vi "BenchmarkSorting.vi"() -> ()   [LabVIEW 2014]
panel:
  out "Bubble Sort(ms)":u32
  out "Insertion Sort(ms)":u32
  out "Selection Sort(ms)":u32
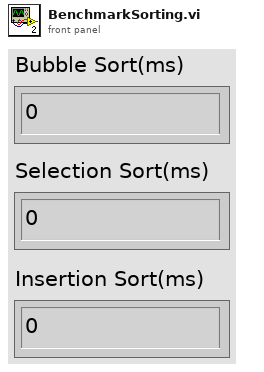
[diagram p1: front panel]
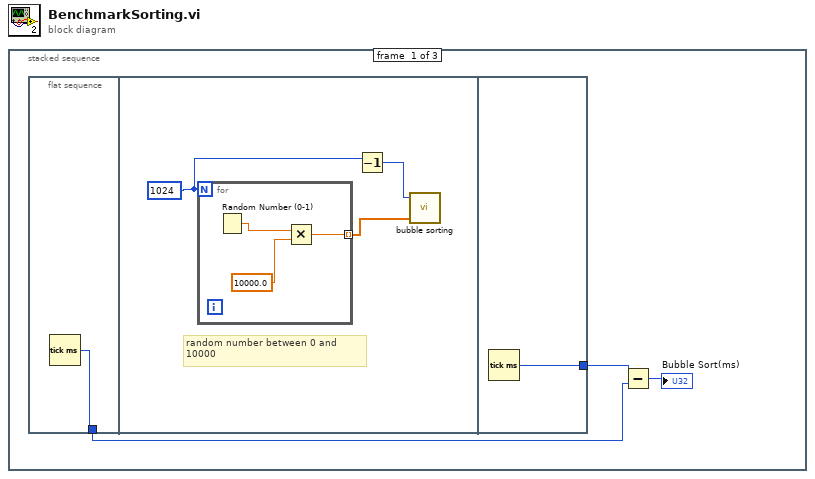
[diagram p0: block diagram]
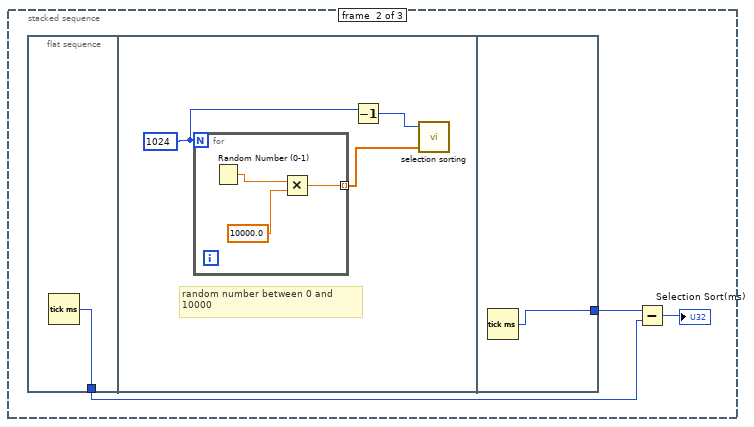
[diagram p2: hidden frame]
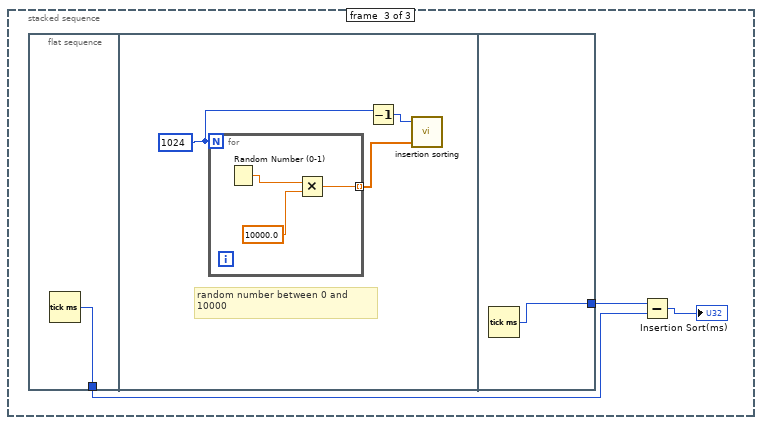
[diagram p3: hidden frame]
diagram:
  n1 = stacked-sequence {
    frame #0 {
      n2 = flat-sequence {
        tunnel: [w4] -> _
        tunnel: [w4] -> w2
        tunnel: [w11] -> w3
        frame #0 {
          n3 = Tick Count (ms)() -> (millisecond timer value=w4:u32)
        }
        frame #1 {
          w7 = 1024
          # "random number between 0 and\n10000"
          n4 = for {
            N: w7 -> [_]
            tunnel: [w8] -> w5 mode=indexing
            n5 = Random Number (0-1)() -> (number: 0 to 1=w10:dbl)
            n6 = Multiply(x=w10, y=10000.0) -> (x*y=w8:dbl)
          }
          n7 = Decrement(x=w7) -> (x-1=w6:i32)
          n8 = call "bubble sorting.vi"("value between1~10000"=w5, "N numbers"=w6) -> ()  [unwired: 3 in]
        }
        frame #2 {
          n9 = Tick Count (ms)() -> (millisecond timer value=w11:u32)
        }
      }
      n10 = Subtract(x=w3, y=w2) -> (x-y=→"Bubble Sort(ms)":u32)
    }
    frame #1 {
      n11 = flat-sequence {
        tunnel: [w15] -> w13
        tunnel: [w22] -> w14
        frame #0 {
          n12 = Tick Count (ms)() -> (millisecond timer value=w15:u32)
        }
        frame #1 {
          w18 = 1024
          # "random number between 0 and\n10000"
          n13 = for {
            N: w18 -> [_]
            tunnel: [w19] -> w16 mode=indexing
            n14 = Random Number (0-1)() -> (number: 0 to 1=w21:dbl)
            n15 = Multiply(x=w21, y=10000.0) -> (x*y=w19:dbl)
          }
          n16 = Decrement(x=w18) -> (x-1=w17:i32)
          n17 = call "selection sorting.vi"("values between 1~10000"=w16, "N numbers"=w17) -> ()  [unwired: 3 in]
        }
        frame #2 {
          n18 = Tick Count (ms)() -> (millisecond timer value=w22:u32)
        }
      }
      n19 = Subtract(x=w14, y=w13) -> (x-y=→"Selection Sort(ms)":u32)
    }
    frame #2 {
      n20 = flat-sequence {
        tunnel: [w26] -> w24
        tunnel: [w33] -> w25
        frame #0 {
          n21 = Tick Count (ms)() -> (millisecond timer value=w26:u32)
        }
        frame #1 {
          w29 = 1024
          # "random number between 0 and\n10000"
          n22 = for {
            N: w29 -> [_]
            tunnel: [w30] -> w27 mode=indexing
            n23 = Random Number (0-1)() -> (number: 0 to 1=w32:dbl)
            n24 = Multiply(x=w32, y=10000.0) -> (x*y=w30:dbl)
          }
          n25 = Decrement(x=w29) -> (x-1=w28:i32)
          n26 = call "insertion sorting.vi"("values between 1~10000"=w27, "N numbers"=w28) -> ()  [unwired: 3 in]
        }
        frame #2 {
          n27 = Tick Count (ms)() -> (millisecond timer value=w33:u32)
        }
      }
      n28 = Subtract(x=w25, y=w24) -> (x-y=→"Insertion Sort(ms)":u32)
    }
  }
